vi "setpointprofileToWaveform.vi"(7 "Time Stamp":timestamp, 9 "Room Temp Offset":dbl, 10 "setpoint profile":cluster{"time (s)":dbl, "setpoint":dbl}[](array[cluster])) -> (2 "Waveform":waveform(dbl))   [LabVIEW 2018]
panel:
  out "sps":dbl[](array[numeric])
  out "dY":dbl[](array[numeric])
  out "dt":dbl[](array[numeric])
  out "slope":dbl[](array[numeric])
  out "Indexed Slopes":dbl[](array[numeric])
  out "Array":dbl[](array[numeric])
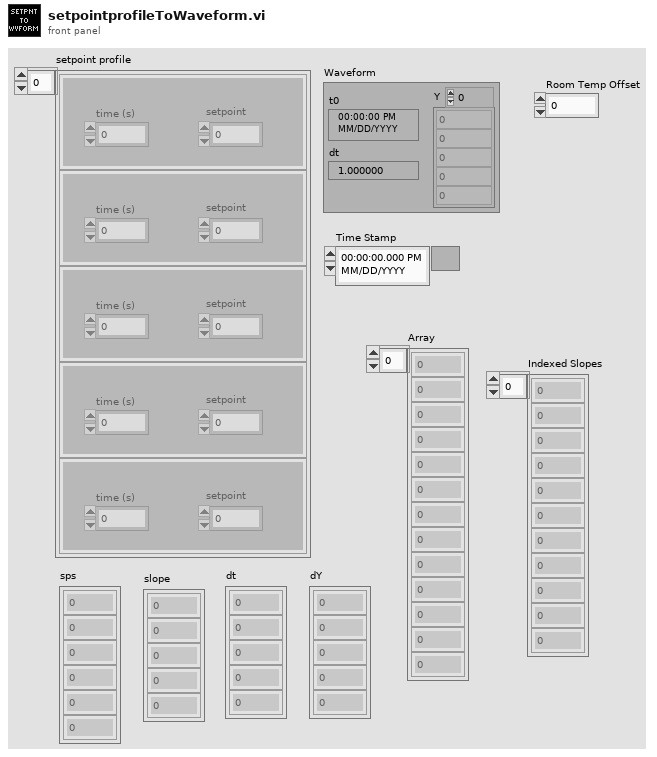
[diagram p1: front panel]
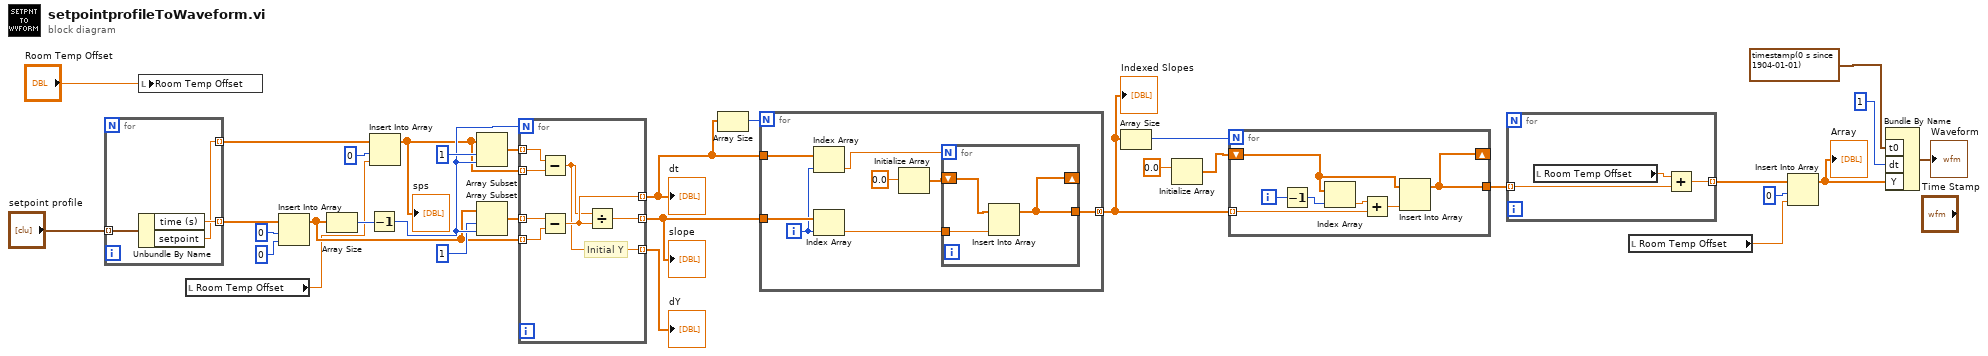
[diagram p0: block diagram]
diagram:
  n1 = for {
    tunnel: "setpoint profile" -> [w35] mode=indexing
    tunnel: [w34] -> w21 mode=indexing
    tunnel: [w33] -> w23 mode=indexing
    n2 = Unbundle By Name(w35) -> ("time (s)"=w34:dbl, "setpoint"=w33:dbl)
  }
  n3 = local write "Room Temp Offset"("Room Temp Offset") -> ()
  n4 = local read "Room Temp Offset"() -> (w17:dbl)
  n5 = Insert Into Array(array=w21, index=0, new element=0) -> (w20:dbl[])
  n6 = Array Size(array=w20) -> (size(s)=w31:i32)
  n7 = Decrement(x=w31) -> (x-1=w27:i32)
  n8 = Insert Into Array(array=w23, index=0, new element=w17) -> (w4:dbl[])
  "sps" <- w4
  n9 = Array Subset(array=w4, index=1, length=w27) -> (w29:dbl[])
  n10 = Array Subset(array=w20, index=1, length=w27) -> (w28:dbl[])
  n11 = for {
    N: w27 -> [_]
    tunnel: w20 -> [w41] mode=indexing
    tunnel: w4 -> [w39] mode=indexing
    tunnel: w29 -> [w40] mode=indexing
    tunnel: w28 -> [w42] mode=indexing
    tunnel: [w36] -> w19 mode=indexing
    tunnel: [w38] -> w15 mode=indexing
    tunnel: [w37] -> w16 mode=indexing
    # "Initial Y"
    n12 = Subtract(x=w40, y=w39) -> (x-y=w36:dbl)
    n13 = Subtract(x=w42, y=w41) -> (x-y=w37:dbl)
    n14 = Divide(x=w36, y=w37) -> (x/y=w38:dbl)
  }
  "slope" <- w15
  "dt" <- w16
  "dY" <- w19
  n15 = Array Size(array=w16) -> (size(s)=w14:i32)
  n16 = for {
    N: w14 -> [_]
    tunnel: w16 -> [w50]
    tunnel: w15 -> [w48]
    tunnel: [w45] -> w12 mode=concatenating
    i -> [w47]
    n17 = Index Array(array=w50, index=w47) -> (element=w49:dbl)
    n18 = Index Array(array=w48, index=w47) -> (element=w46:dbl)
    n19 = Initialize Array(0.0) -> (w44:dbl[])  [unwired: 1 in]
    n20 = for {
      N: w49 -> [_]
      tunnel: w46 -> [w53]
      tunnel: [w52] -> w45
      shift-right: [w52] -> _
      shift-left: w44 -> [w51]
      n21 = Insert Into Array(array=w51, new element=w53) -> (w52:dbl[])  [unwired: 1 in]
    }
  }
  "Indexed Slopes" <- w12
  n22 = Array Size(array=w12) -> (size(s)=w13:i32)
  n23 = Initialize Array(0.0) -> (w1:dbl[])  [unwired: 1 in]
  n24 = for {
    N: w13 -> [_]
    tunnel: w12 -> [w60] mode=indexing
    tunnel: [w55] -> w11
    shift-right: [w55] -> _
    shift-left: w1 -> [w54]
    i -> [w57]
    n25 = Decrement(x=w57) -> (x-1=w56:i32)
    n26 = Index Array(array=w54, index=w56) -> (element=w58:dbl)
    n27 = Add(x=w58, y=w60) -> (x+y=w59:dbl)
    n28 = Insert Into Array(array=w54, new element=w59) -> (w55:dbl[])  [unwired: 1 in]
  }
  n29 = for {
    tunnel: w11 -> [w62] mode=indexing
    tunnel: [w61] -> w8 mode=indexing
    n30 = local read "Room Temp Offset"() -> (w63:dbl)
    n31 = Add(x=w63, y=w62) -> (x+y=w61:dbl)
  }
  n32 = local read "Room Temp Offset"() -> (w10:dbl)
  n33 = Insert Into Array(array=w8, index=0, new element=w10) -> (w6:dbl[])
  "Array" <- w6
  n34 = Bundle By Name("t0"=timestamp(0 s since 1904-01-01), "dt"=1, "Y"=w6) -> (→"Waveform":waveform(dbl))  [unwired: 1 in]
